vi "Get Msgs.vi"(11 "TEMPLATE Actor in":refnum<class "TEMPLATE Actor.lvclass">) -> (2 "Msgs":T1)   [LabVIEW 2020, in "_Template.lvlib" / "Templates.lvlib" / "TEMPLATE Actor.lvlib" / "TEMPLATE Actor.lvclass"]
uses:
  TEMPLATE Actor.lvclass
  jettl/jettl/Actor/Msg Set.ctl
  jettl/jettl/Msg/Msg.lvclass
  TEMPLATE Actor.lvclass/TEMPLATE Actor.ctl
  jettl/jettl/Actor/Actor.lvlib
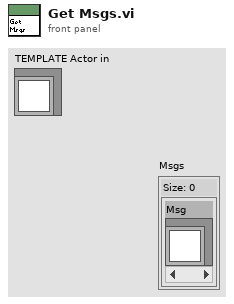
[diagram p1: front panel]
types:
  T1 = typedef "jettl.lvlib/Actor.lvlib/Msg Set.ctl" = set{refnum<class "Msg.lvclass">}
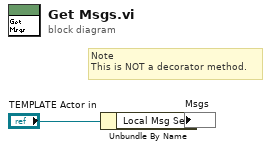
[diagram p0: block diagram]
diagram:
  # "Note\nThis is NOT a decorator method."
  n1 = Unbundle By Name("TEMPLATE Actor in") -> ("Local Msg Set"=→"Msgs":T1)
